vi "RS232ComPort ReadPortInfo.vi"(8 "error in (no error)":errorcluster, 9 "Channel":i32, 11 "RS232ComPort in":refnum<class "RS232ComPort.lvclass">) -> (0 "error out":errorcluster, 2 "Status":i8, 3 "RS232ComPort out":refnum<class "RS232ComPort.lvclass">)   [LabVIEW 2018, in "RS232ComPort.lvclass"]
doc: "Channel status\n-1 | Laser\n0 | Not in used so far\n0..127 | # of device initialising with @"
uses:
  RS232ComPort.lvclass
  RS232ComPort.lvclass/RS232ComPort.ctl
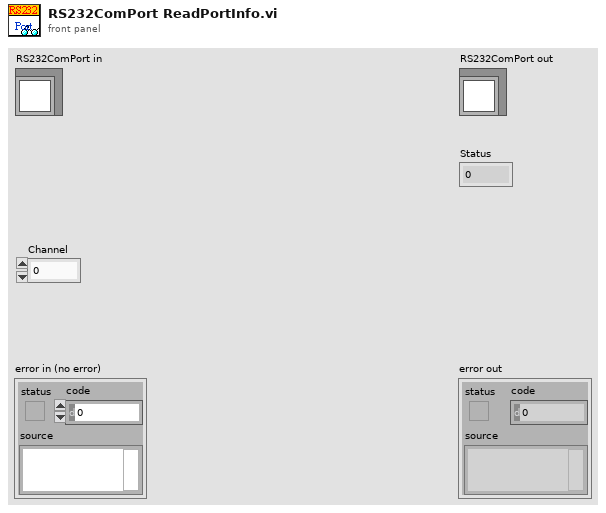
[diagram p1: front panel]
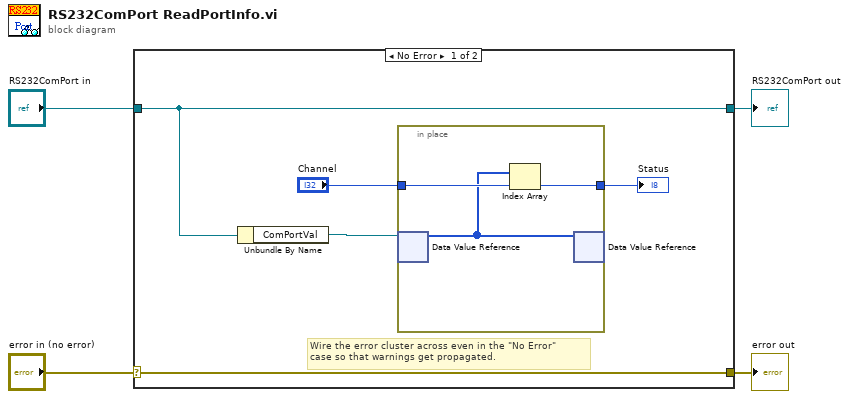
[diagram p0: block diagram]
diagram:
  n1 = case shown="No Error" "error in (no error)" {
    selector: "error in (no error)" -> [w9 w14]
    tunnel: [w9 w14] -> w3
    tunnel: [w8 w13] -> w1
    tunnel: "RS232ComPort in" -> [w8 w13]
    frame No Error {
      # "Wire the error cluster across even in the \"No Error\"\ncase so that warnings get propagated."
      n2 = Unbundle By Name(w8) -> ("ComPortVal"=w7:refnum<data-value>)
      n3 = in-place {
        in-place-border: "Channel" -> [w12]
        in-place-border: [w10] -> w5
        n4 = in-place-dvr #1(w7) -> (w11:i8[])  [unwired: 1 out]
        n5 = Index Array(array=w11, index=w12) -> (element=w10:i8)
        n6 = in-place-dvr #1(w11) -> ()  [unwired: 2 out]
      }
      "Status" <- w5
    }
    frame Error {
    }
  }
  "error out" <- w3
  "RS232ComPort out" <- w1
